vi "CMD_HOME.vi"(6 "Gantry in":refnum<class "Gantry.lvclass">, 8 "error in (no error)":errorcluster, 10 "Arguments":string[](array[string]), 11 "gScript Interpreter in":refnum<class "gScript Interpreter.lvclass">) -> (0 "error out":errorcluster, 3 "gScript Interpreter out":refnum<class "gScript Interpreter.lvclass">, 4 "Gantry out":refnum<class "Gantry.lvclass">)   [LabVIEW 2017, in "gScript Interpreter.lvclass"]
uses:
  gScript Interpreter.lvclass
  Shared Components/Gantry Class/Gantry.lvclass
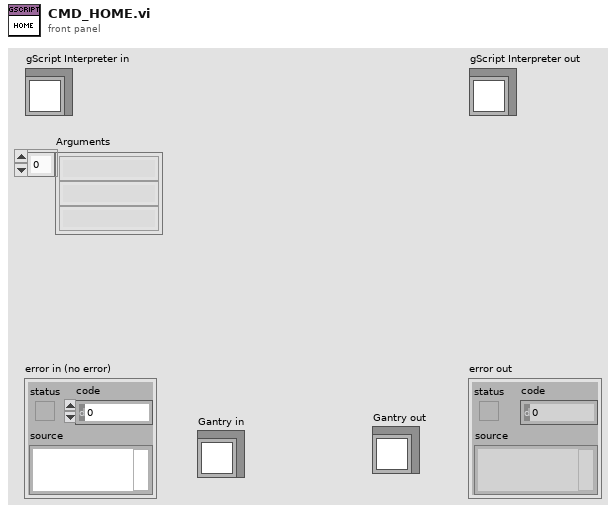
[diagram p1: front panel]
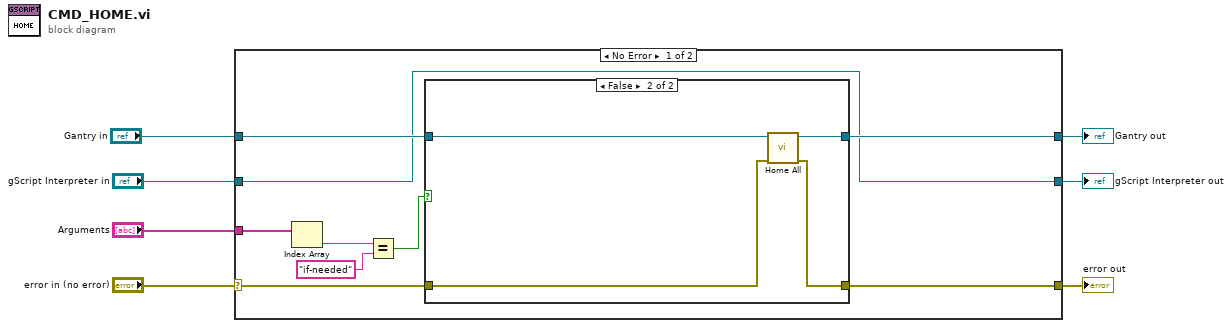
[diagram p0: block diagram]
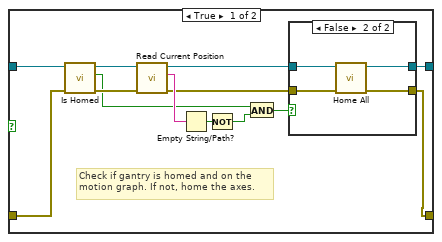
[diagram p2: hidden frame]
diagram:
  n1 = case shown="No Error" "error in (no error)" {
    selector: "error in (no error)" -> [w14 w42]
    tunnel: [w13 w42] -> w6
    tunnel: [w8 w41] -> w4
    tunnel: "gScript Interpreter in" -> [w8 w41]
    tunnel: "Arguments" -> [w12 _]
    tunnel: "Gantry in" -> [w16 w40]
    tunnel: [w15 w40] -> w1
    frame No Error {
      n2 = Index Array(array=w12) -> (element=w11:string)  [unwired: 1 in]
      n3 = Equal?(x=w11, y="if-needed") -> (x = y?=w9:bool)
      n4 = case shown="False" w9 {
        tunnel: w16 -> [w29 w39]
        tunnel: [w20 w38] -> w15
        tunnel: w14 -> [w27 w37]
        tunnel: [w17 w36] -> w13
        frame True {
          # "Check if gantry is homed and on the\nmotion graph. If not, home the axes."
          n5 = call "Is Homed.vi"("error in (no error)"=w27, "Gantry in"=w29) -> ("error out"=w26:errorcluster, "homed?"=w23:bool, "Gantry out"=w28:refnum<class "Gantry.lvclass">)  [unwired: 7 in]
          n6 = call-dynamic "Read Current Position.vi"("error in"=w26, "Gantry in"=w28) -> ("error out"=w18:errorcluster, "Current Position"=w25:string, "Gantry out"=w21:refnum<class "Gantry.lvclass">)  [unwired: 7 in]
          n7 = Empty String/Path?(string/path=w25) -> (empty?=w24:bool)
          n8 = Not(x=w24) -> (.not. x?=w22:bool)
          n9 = And(x=w23, y=w22) -> (x .and. y?=w19:bool)
          n10 = case shown="False" w19 {
            tunnel: w21 -> [w31 w35]
            tunnel: [w31 w34] -> w20
            tunnel: w18 -> [w30 w33]
            tunnel: [w30 w32] -> w17
            frame True {
            }
            frame False {
              n11 = call "Home All.vi"("error in (no error)"=w33, "Gantry in"=w35) -> ("error out"=w32:errorcluster, "Gantry out"=w34:refnum<class "Gantry.lvclass">)  [unwired: 8 in]
            }
          }
        }
        frame False {
          n12 = call "Home All.vi"("error in (no error)"=w37, "Gantry in"=w39) -> ("error out"=w36:errorcluster, "Gantry out"=w38:refnum<class "Gantry.lvclass">)  [unwired: 8 in]
        }
      }
    }
    frame Error {
    }
  }
  "error out" <- w6
  "gScript Interpreter out" <- w4
  "Gantry out" <- w1
